vi "SubVI_Convert_Impedances.vi"(8 "error in (no error)":errorcluster, 10 "Weight Array":i32[](array[numeric]), 11 "Raw Impedances in":T1) -> (0 "error out":errorcluster, 3 "Converted Impedances Out":T2)   [LabVIEW 2020]
uses:
  <extravilib>/ChannelInstances/Lossy Stream-a[.](dbl)/)Channel.ctl
  <extravilib>/ChannelInstances/Lossy Stream-a[.](u8)/)Channel.ctl
  <extravilib>/ChannelInstances/Lossy Stream-a[.](u8)/EndpointRead.vi
  <extravilib>/ChannelInstances/Lossy Stream-a[.](dbl)/Endpoint.vi
  <extravilib>/ChannelInstances/Lossy Stream-a[.](u8)/)Channel.vi
  <resource>/ChannelSupport/_ChannelSupport/WaitIfNeeded.vi
  <extravilib>/ChannelInstances/Lossy Stream-a[.](dbl)/)Channel.vi
  <extravilib>/ChannelInstances/Lossy Stream-a[.](u8).lvlib
  <extravilib>/ChannelInstances/Lossy Stream-a[.](dbl).lvlib
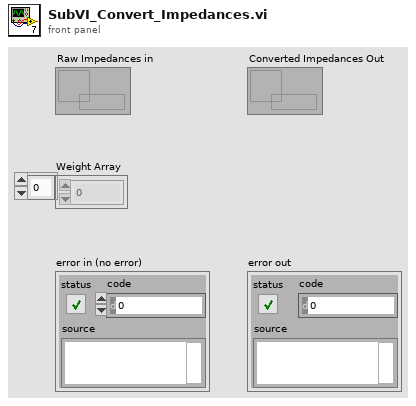
[diagram p1: front panel]
types:
  T1 = typedef "Lossy Stream-a[.](u8).lvlib/)Channel.ctl" = refnum<queue>
  T2 = typedef "Lossy Stream-a[.](dbl).lvlib/)Channel.ctl" = refnum<queue>
  T3 = typedef "LVDateTimeRec.ctl" = cluster{"fractional second":dbl, "second":i32, "minute":i32, "hour":i32, "day of month":i32, "month":i32, "year":i32, "day of week":i32, "day of year":i32, "DST":i32}
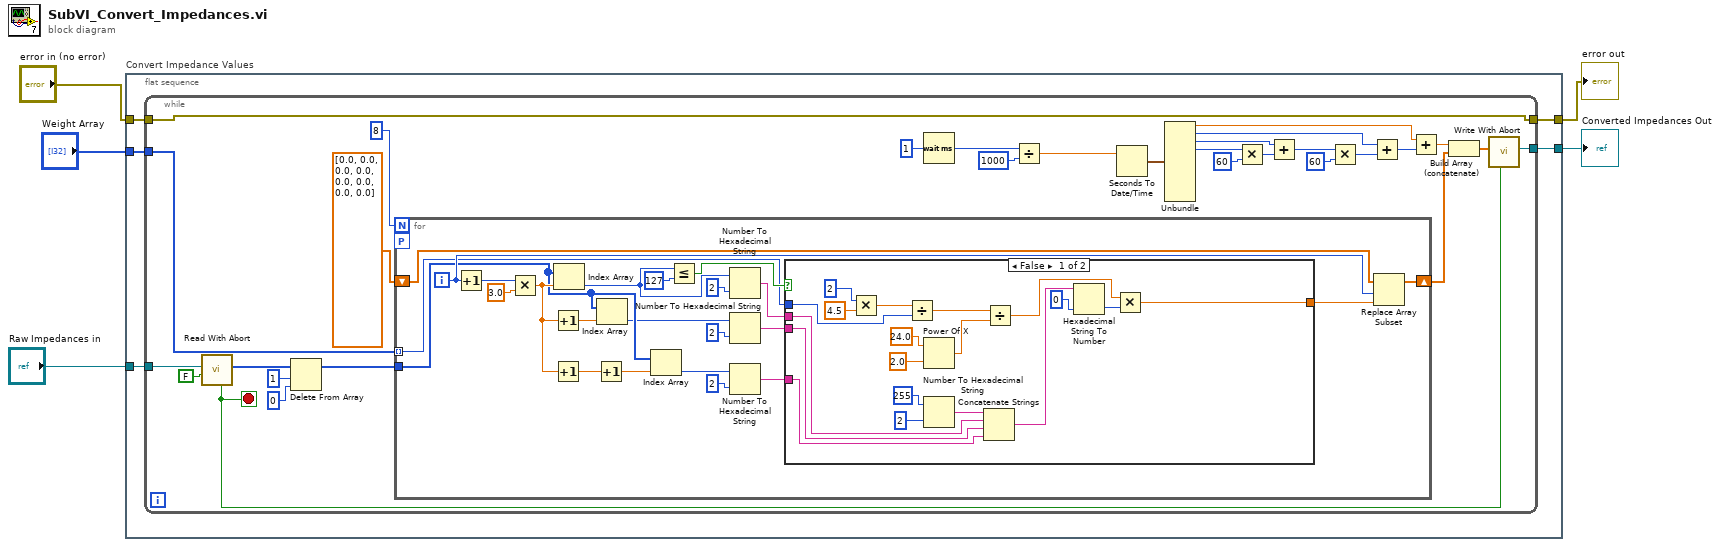
[diagram p0: block diagram]
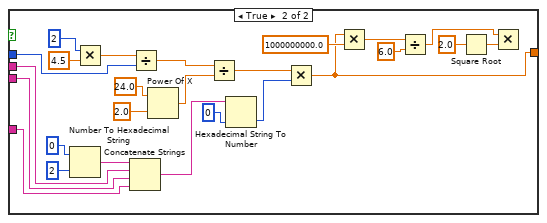
[diagram p2: hidden frame]
diagram:
  n1 = flat-sequence "Convert Impedance Values" {
    tunnel: "Raw Impedances in" -> [w10]
    tunnel: "Weight Array" -> [w9]
    tunnel: [w8] -> w3
    tunnel: [w7] -> w4
    tunnel: "error in (no error)" -> [w6]
    frame #0 {
      n2 = while {
        tunnel: w10 -> [w36]
        tunnel: w9 -> [w33]
        tunnel: w6 -> [w31]
        tunnel: [w31] -> w8
        tunnel: [w14] -> w7
        stop <- w11 stop-if-true
        n3 = call <extravilib>:"Read With Abort.vi"("abort"=FALSE, "channel"=w36) -> ("element"=w34:u8[], "aborted?"=w11:bool)  [unwired: 3 in, 5 out]
        n4 = Delete From Array(array=w34, length=1, index=0) -> (array with subset deleted=w32:u8[])  [unwired: 1 out]
        n5 = for {
          N: 8 -> [_]
          shift-right: [w46] -> w12
          shift-left: dbl[] [0.0, 0.0, 0.0, 0.0, 0.0, 0.0, 0.0, 0.0] -> [w47]
          tunnel: w32 -> [w45]
          tunnel: w33 -> [w41] mode=indexing
          workers-P: _ -> [_]
          i -> [w48]
          n6 = Increment(x=w48) -> (x+1=w54:i32)
          n7 = Multiply(x=w54, y=3.0) -> (x*y=w53:dbl)
          n8 = Increment(x=w53) -> (x+1=w50:dbl)
          n9 = Increment(x=w53) -> (x+1=w51:dbl)
          n10 = Index Array(array=w45, index=w53) -> (element=w42:u8)
          n11 = Increment(x=w51) -> (x+1=w52:dbl)
          n12 = Index Array(array=w45, index=w50) -> (element=w43:u8)
          n13 = Index Array(array=w45, index=w52) -> (element=w44:u8)
          n14 = Less Or Equal?(x=w42, y=u8 127) -> (x <= y?=w62:bool)
          n15 = Number To Hexadecimal String(1:i16 2 ("width (-)"), 2:w42) -> (0:w59:string)
          n16 = Number To Hexadecimal String(1:i16 2 ("width (-)"), 2:w43) -> (0:w60:string)
          n17 = Number To Hexadecimal String(1:i16 2 ("width (-)"), 2:w44) -> (0:w61:string)
          n18 = case shown="False" w62 {
            tunnel: w61 -> [w73 w97]
            tunnel: w60 -> [w74 w96]
            tunnel: w59 -> [w75 w95]
            tunnel: [w64 w83] -> w49
            tunnel: w41 -> [w65 w90]
            frame False {
              n19 = Multiply(x=2, y=4.5) -> (x*y=w80:dbl)
              n20 = Divide(x=w80, y=w65) -> (x/y=w77:dbl)
              n21 = Power Of X(1:2.0 ("x"), 2:24.0 ("y")) -> (0:w76:dbl)
              n22 = Number To Hexadecimal String(1:i16 2 ("width (-)"), 2:255) -> (0:w71:string)
              n23 = Concatenate Strings(w71, w75, w74, w73) -> (w68:string)
              n24 = Divide(x=w77, y=w76) -> (x/y=w70:dbl)
              n25 = Hexadecimal String To Number(string=w68, default (0uL)=0 ("default (0 U32)")) -> (number=w67:i32)  [unwired: 1 in, 1 out]
              n26 = Multiply(x=w70, y=w67) -> (x*y=w64:dbl)
            }
            frame True {
              n27 = Number To Hexadecimal String(1:i16 2 ("width (-)"), 2:0) -> (0:w99:string)
              n28 = Multiply(x=2, y=4.5) -> (x*y=w105:dbl)
              n29 = Concatenate Strings(w99, w95, w96, w97) -> (w93:string)
              n30 = Divide(x=w105, y=w90) -> (x/y=w102:dbl)
              n31 = Power Of X(1:2.0 ("x"), 2:24.0 ("y")) -> (0:w101:dbl)
              n32 = Divide(x=w102, y=w101) -> (x/y=w98:dbl)
              n33 = Hexadecimal String To Number(string=w93, default (0uL)=0 ("default (0 U32)")) -> (number=w94:i32)  [unwired: 1 in, 1 out]
              n34 = Multiply(x=w98, y=w94) -> (x*y=w83:dbl)
              n35 = Multiply(x=w83, y=1000000000.0) -> (x*y=w88:dbl)
              n36 = Divide(x=w88, y=6.0) -> (x/y=w86:dbl)
              n37 = Square Root(x=2.0) -> (sqrt(x)=w84:dbl)
              n38 = Multiply(x=w86, y=w84) -> ()  [unwired: 1 out]
            }
          }
          n39 = Replace Array Subset(array=w47, new element=w49, index=w48) -> (w46:dbl[])
        }
        n40 = Wait (ms)(milliseconds to wait=u32 1) -> (millisecond timer value=w27:u32)
        n41 = Divide(x=w27, y=u32 1000) -> (x/y=w28:dbl)
        n42 = Seconds To Date/Time(time stamp (now)=w28) -> (date time rec=w26:T3)  [unwired: 1 in]
        n43 = Unbundle(w26) -> ("fractional second"=w16:dbl, "second"=w17:i32, "minute"=w19:i32, "hour"=w21:i32)  [unwired: 6 out]
        n44 = Multiply(x=w21, y=60) -> (x*y=w25:i32)
        n45 = Add(x=w19, y=w25) -> (x+y=w24:i32)
        n46 = Multiply(x=w24, y=60) -> (x*y=w23:i32)
        n47 = Add(x=w17, y=w23) -> (x+y=w22:i32)
        n48 = Add(x=w16, y=w22) -> (x+y=w13:dbl)
        n49 = Build Array (concatenate)(w13, w12) -> (w15:dbl[])
        n50 = call <extravilib>:"Write With Abort.vi"("abort"=w11, "element"=w15) -> ("channel"=w14:T2)  [unwired: 6 in, 3 out]
      }
    }
  }
  "Converted Impedances Out" <- w4
  "error out" <- w3
